vi "File Counter.vi"(11 "Error in":errorcluster, 13 "Operations":T1(ring)) -> (4 "Count":i32, 6 "Count":string, 15 "Error out":errorcluster)   [LabVIEW 2021]
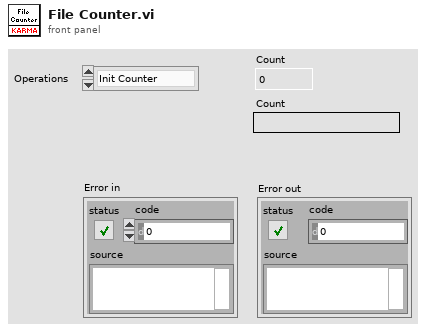
[diagram p1: front panel]
types:
  T1 = enum16{"Init Counter", "Read Last Value", "Write Last Value", "Reset Counter", "Increment by 1", "Decrement by 1", "Get Current Count"}
  T2 = enum16{"open", "replace", "create", "open or create", "replace or create", "replace or create with confirmation"}
  T3 = typedef "Paths.ctl" = cluster{"Configuration":path, "Event Logs":path, "Error Logs":path, "Macros":path, "Camera Settings":path, "Settings.ini":path, "UserInfo.bin":path, "TimeStamp File":path, "FileCounter.txt":path, "FFC Images":path, "Calibration.txt":path, "Bright Images - FFC":path, "Dark Images - FFC":path, "Last FFC Time File":path, "BG Subtraction Folder":path, "BG Mask":path, "LUTs Folder":path}
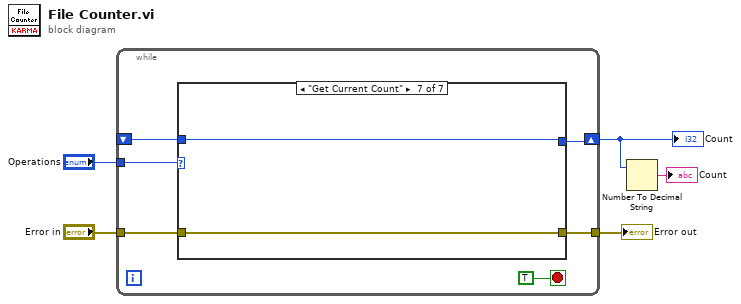
[diagram p0: block diagram]
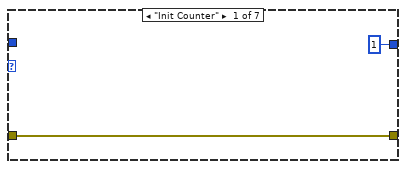
[diagram p2: hidden frame]
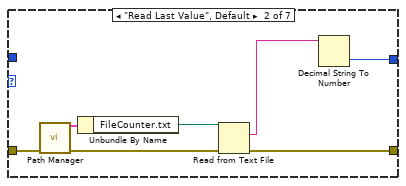
[diagram p3: hidden frame]
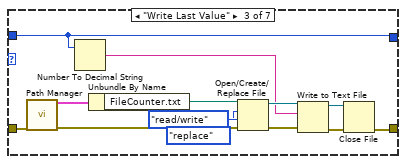
[diagram p4: hidden frame]
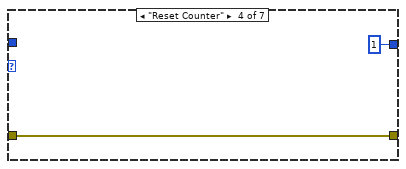
[diagram p5: hidden frame]
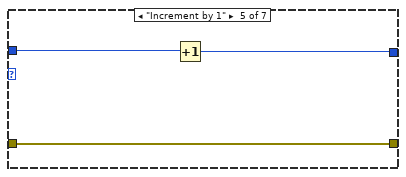
[diagram p6: hidden frame]
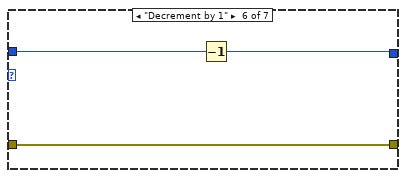
[diagram p7: hidden frame]
diagram:
  n1 = while {
    shift-right: [w10] -> w2
    shift-left: _ -> [w8]
    tunnel: "Operations" -> [w9]
    tunnel: "Error in" -> [w7]
    tunnel: [w6] -> w3
    stop <- TRUE stop-if-true
    n2 = case shown="\"Get Current Count\"" w9 {
      tunnel: [1 w15 w22 1 w37 w40 w43] -> w10
      tunnel: w8 -> [_ _ w22 _ w38 w41 w43]
      tunnel: w7 -> [w12 w20 w28 w34 w36 w39 w42]
      tunnel: [w12 w14 w24 w34 w36 w39 w42] -> w6
      frame "Init Counter" {
      }
      frame "Read Last Value", Default {
        n3 = call "Path Manager.vi"("error in (no error)"=w20) -> ("Cluster"=w18:T3, "Error out"=w19:errorcluster)  [unwired: 13 in]
        n4 = Unbundle By Name(w18) -> ("FileCounter.txt"=w17:path)
        n5 = Read from Text File(file (use dialog)=w17, error in=w19) -> (text=w16:string, error out=w14:errorcluster)  [unwired: 2 in, 2 out]
        n6 = Decimal String To Number(string=w16) -> (number=w15:i32)  [unwired: 2 in, 1 out]
      }
      frame "Write Last Value" {
        n7 = call "Path Manager.vi"("error in (no error)"=w28) -> ("Cluster"=w31:T3, "Error out"=w33:errorcluster)  [unwired: 13 in]
        n8 = Number To Decimal String(number=w22) -> (decimal integer string=w21:string)  [unwired: 1 in]
        n9 = Unbundle By Name(w31) -> ("FileCounter.txt"=w32:path)
        n10 = Open/Create/Replace File(file path (use dialog)=w32, error in=w33, operation (0:open)=T2."replace", access (0:read/write)=enum16{"read/write", "read-only", "write-only"}."read/write") -> (refnum out=w26:refnum<file>, error out=w27:errorcluster)  [unwired: 2 in, 1 out]
        n11 = Write to Text File(file (use dialog)=w26, text=w21, error in=w27) -> (refnum out=w23:refnum<file>, error out=w25:errorcluster)  [unwired: 1 in, 1 out]
        n12 = Close File(refnum=w23, error in=w25) -> (error out=w24:errorcluster)  [unwired: 1 out]
      }
      frame "Reset Counter" {
      }
      frame "Increment by 1" {
        n13 = Increment(x=w38) -> (x+1=w37:i32)
      }
      frame "Decrement by 1" {
        n14 = Decrement(x=w41) -> (x-1=w40:i32)
      }
      frame "Get Current Count" {
      }
    }
  }
  "Error out" <- w3
  "Count" <- w2
  n15 = Number To Decimal String(number=w2) -> (decimal integer string=→"Count":string)  [unwired: 1 in]
